vi "Loops als Cluster.vi"(8 "error in (no error)":errorcluster caption="Fehler (Eingang, kein Fehler)", 11 "Steuerung PNS Eingang":refnum<class "Steuerung PNS.lvclass">) -> (0 "error out":errorcluster caption="Fehler (Ausgang)", 2 "LoopGeraetekennung":T1, 3 "Steuerung PNS Ausgang":refnum<class "Steuerung PNS.lvclass">)   [LabVIEW 2020, in "Steuerung PNS.lvclass"]
doc: "Gibt das Array mit den Loopnamen in der jeweiligen Sprache gemeinsam mit der Gerätetype als Cluster zurück.\n(zum schreiben in die FGV Loopkennung)\nRIW"
uses:
  Steuerung PNS.lvclass
  PNS/PNS Geraetekennung.ctl
  PNS/PNS.lvlib
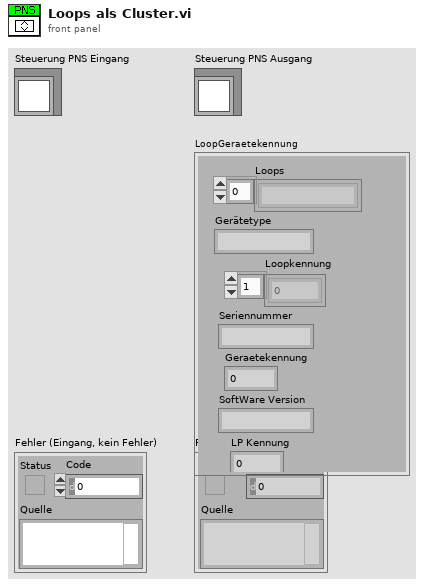
[diagram p1: front panel]
types:
  T1 = typedef "PNS.lvlib/PNS Geraetekennung.ctl" = cluster{"Loops":string[], "Gerätetype":string, "Loopkennung":u16[], "Seriennummer":string, "Geraetekennung":u16, "SoftWare Version":string, "LP Kennung":u16}
  T2 = cluster{"Loops":string[], "Geraetetype":string, "Loopkennung":u16[], "Seriennummer":string, "Geraetekennung":u16, "SoftWare Version":string, "LP Kennung":u16}
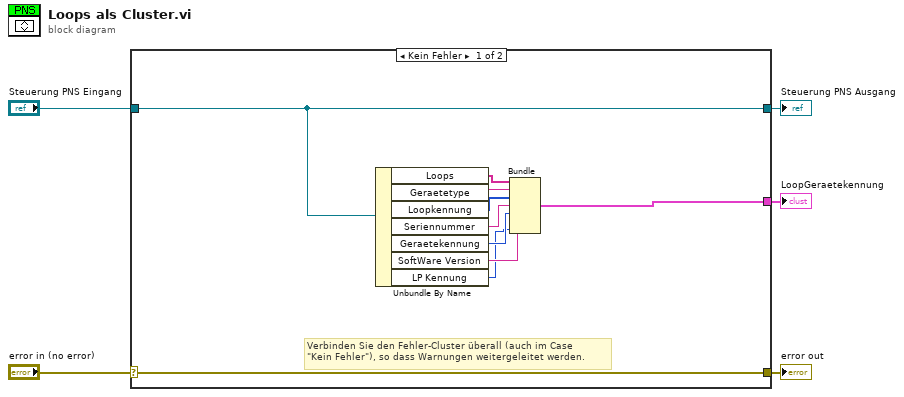
[diagram p0: block diagram]
diagram:
  n1 = case shown="Kein Fehler" "error in (no error)" {
    selector: "error in (no error)" -> [w15 w17]
    tunnel: [w15 w17] -> w4
    tunnel: [w14 w16] -> w2
    tunnel: "Steuerung PNS Eingang" -> [w14 w16]
    tunnel: [w11 _] -> w1
    frame No Error {
      # "Verbinden Sie den Fehler-Cluster überall (auch im Case\n\"Kein Fehler\"), so dass Warnungen weitergeleitet werden."
      n2 = Unbundle By Name(w14) -> ("Loops"=w13:string[], "Geraetetype"=w12:string, "Loopkennung"=w10:u16[], "Seriennummer"=w9:string, "Geraetekennung"=w8:u16, "SoftWare Version"=w7:string, "LP Kennung"=w6:u16)
      n3 = Bundle("Loops"=w13, "Geraetetype"=w12, "Loopkennung"=w10, "Seriennummer"=w9, "Geraetekennung"=w8, "SoftWare Version"=w7, "LP Kennung"=w6) -> (w11:T2)  [unwired: 1 in]
    }
    frame Error {
    }
  }
  "error out" <- w4
  "Steuerung PNS Ausgang" <- w2
  "LoopGeraetekennung" <- w1
